vi "FlpLib ThreePhasePLL 3.vi"(0 "Vq":sgl, 1 "PLLgains":T3 {"proportional gain" step=0.125}, 3 "PLLrange":T2={"output high (Inf)"=inf, "output low (-Inf)"=-inf}, 5 "dT":sgl, 9 "GridExpectedFreq":sgl, 11 "Phase In":sgl, 12 "reset":bool) -> (4 "gridFrequency":sgl, 10 "PLLactions":T1, 15 "Phase Out":sgl)   [LabVIEW 2017]
uses:
  <vilib>/rvi/Analysis/control/PID/Typedef/niFpgaPID_PIGains.ctl
  <vilib>/rvi/Analysis/control/PID/Typedef/niFpgaPID_OutputRange.ctl
  <vilib>/rvi/Analysis/control/PID/Typedef/niFpgaPID_PIActions.ctl
  <vilib>/rvi/Analysis/control/PID/Typedef/niFpgaPID_PIState.ctl
  <userlib>/_NI FLP Library/FPGA/outsideSCTL/FlpLib Multiply Shared Instance 3.vi
  Control/PI_Controller/FlpLib PI_Controller 3.vi
  <userlib>/_NI FLP Library/FPGA/outsideSCTL/FlpLib Add Shared Instance 3.vi
  <userlib>/_NI FLP Library/FPGA/outsideSCTL/FlpLib Subtract Shared Instance 3.vi
  <userlib>/_NI FLP Library/FPGA/outsideSCTL/FlpLib Greater Than Shared Instance 3.vi
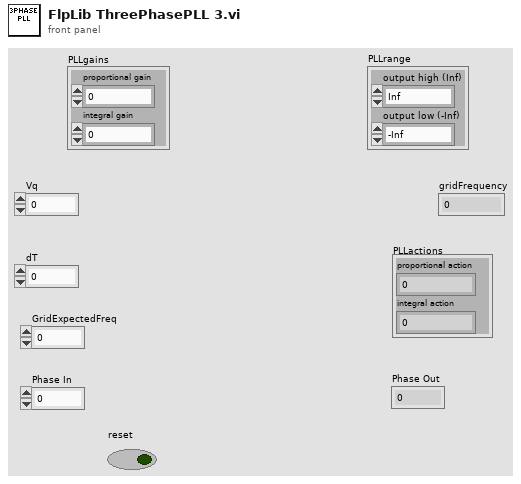
[diagram p1: front panel]
types:
  T1 = typedef "niFpgaPID_PIActions.ctl" = cluster{"proportional action":sgl, "integral action":sgl}
  T2 = typedef "niFpgaPID_OutputRange.ctl" = cluster{"output high (Inf)":sgl, "output low (-Inf)":sgl}
  T3 = typedef "niFpgaPID_PIGains.ctl" = cluster{"proportional gain":sgl, "integral gain":sgl}
  T4 = typedef "niFpgaPID_PIState.ctl" = cluster{"uI(k-1)":sgl, "e(k-1)":sgl, "output (k-1)":sgl}
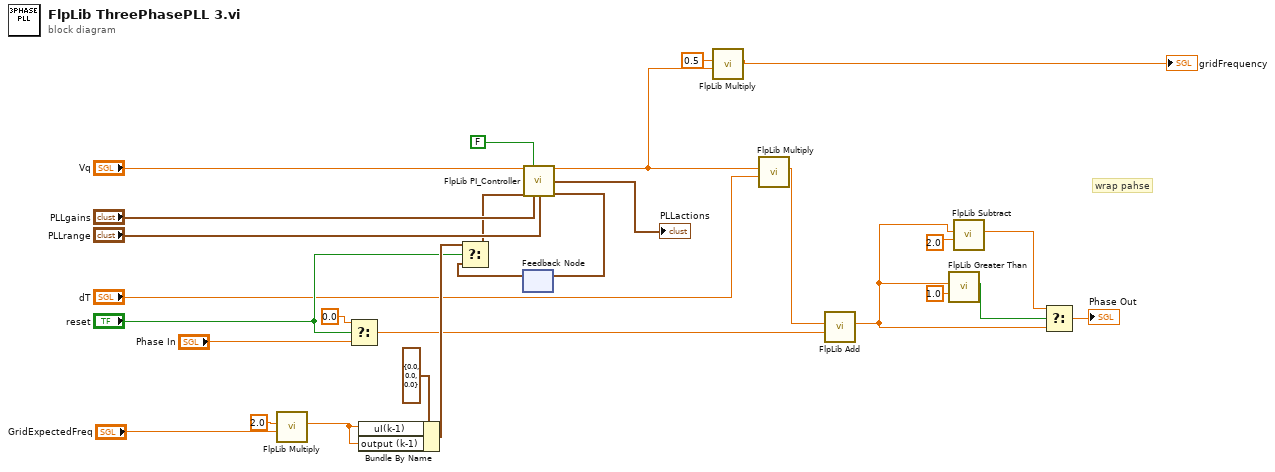
[diagram p0: block diagram]
diagram:
  # "wrap pahse"
  n1 = call-poly <userlib>:"FlpLib Multiply.vi"("y"="GridExpectedFreq", "x"=sgl 2.0) -> ("x*y"=w9:sgl)  [unwired: 5 in]
  n2 = Select(t=sgl 0.0, s="reset", f="Phase In") -> (s? t:f=w7:sgl)
  n3 = Bundle By Name(cluster=T4 {"uI(k-1)"=0.0, "e(k-1)"=0.0, "output (k-1)"=0.0} ("state out"), "uI(k-1)"=w9, "output (k-1)"=w9) -> (w20:T4)
  n4 = feedback #1() -> (w19:T4)  [unwired: 1 in]
  n5 = Select(t=w20, s="reset", f=w19) -> (s? t:f=w18:T4)
  n6 = call-poly "FlpLib PI_Controller.vi"("error"="Vq", "reset? (F)"=FALSE, "state in"=w18, "gains"="PLLgains", "output range"="PLLrange") -> ("output"=w13:sgl, "actions"=→"PLLactions":T1, "state out"=w28:T4)  [unwired: 7 in, 1 out]
  n7 = feedback-in #1(w28) -> ()
  n8 = call-poly <userlib>:"FlpLib Multiply.vi"("y"=w13, "x"=sgl 0.5) -> ("x*y"=→"gridFrequency":sgl)  [unwired: 5 in]
  n9 = call-poly <userlib>:"FlpLib Multiply.vi"("y"="dT", "x"=w13) -> ("x*y"=w8:sgl)  [unwired: 5 in]
  n10 = call-poly <userlib>:"FlpLib Add.vi"("y"=w7, "x"=w8) -> ("x+y"=w5:sgl)  [unwired: 5 in]
  n11 = call-poly <userlib>:"FlpLib Greater Than.vi"("y"=sgl 1.0, "x"=w5) -> ("x > y?"=w24:bool)  [unwired: 5 in]
  n12 = call-poly <userlib>:"FlpLib Subtract.vi"("y"=sgl 2.0, "x"=w5) -> ("x-y"=w4:sgl)  [unwired: 5 in]
  n13 = Select(t=w4, s=w24, f=w5) -> (s? t:f=→"Phase Out":sgl)
